vi "Continuous Output.vi"() -> ()   [LabVIEW 2014]
doc: "This example demonstrates how to continuously re-generate analog output data from a buffer in your computer's memory.\n\nRefer to your device documentation for pinouts and hardware capabilities."
uses:
  <vilib>/Utility/error.llb/DialogType.ctl
  <vilib>/DAQmx/write.llb/DAQmx Write (Analog 1D Wfm NChan NSamp).vi
  <vilib>/DAQmx/create/channels.llb/DAQmx Create Channel (AO-Voltage-Basic).vi
  <vilib>/DAQmx/configure/timing.llb/DAQmx Timing (Sample Clock).vi
  <vilib>/DAQmx/miscellaneous.llb/DAQmx Fill In Error Info.vi
  <resource>/objmgr/daqmx.rc
  <vilib>/measure/NI_MABase.lvlib
panel:
  in  "Output Array":T1(array[cluster])=[{"Waveform Type"=0, "Amplitude"=1.0, "Frequency"=10.0}] {"Frequency" format="%0.2p"; "Amplitude" format="%0.2p"; "Waveform Type" items=["Sine Wave", "Triangle Wave", "Square Wave", "Sawtooth Wave"]}
  in  "Number of Samples":i32=1000
  in  "Stop":bool
  out "Waveform Graph":waveform(dbl)[](graph)=[{"t0"=timestamp(0 s since 1904-01-01), "dt"=0.001, "Y"=[]}]
  in  "Sample Rate":dbl=1000.0
  in  "Sample Clock Source":tag="OnboardClock"
  in  "Max Voltage":dbl=5.0
  in  "Min Voltage":dbl=-5.0
  in  "Physical Channel(s)":tag="Dev1/ao0"
  out "Actual Sample Rate":dbl=1000.0 format="%0.2f"
  # "Channel Settings"
  # "Output"
  # "Timing and Buffer Settings"
  # "Waveform Settings"
  # "The number of elements in the waveform array must equal the number of channels in the task."
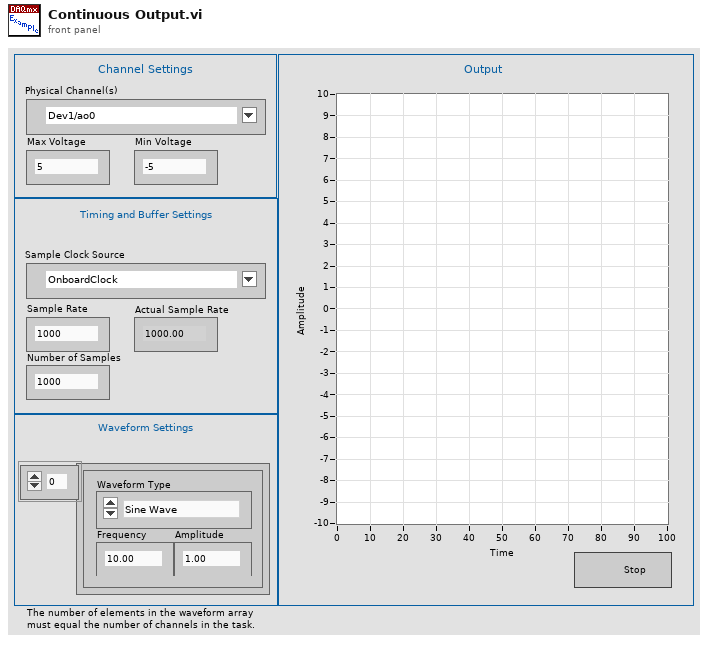
[diagram p1: front panel]
types:
  T1 = cluster{"Waveform Type":u16, "Amplitude":dbl, "Frequency":dbl}[]
  T2 = typedef "DialogType.ctl" = u16
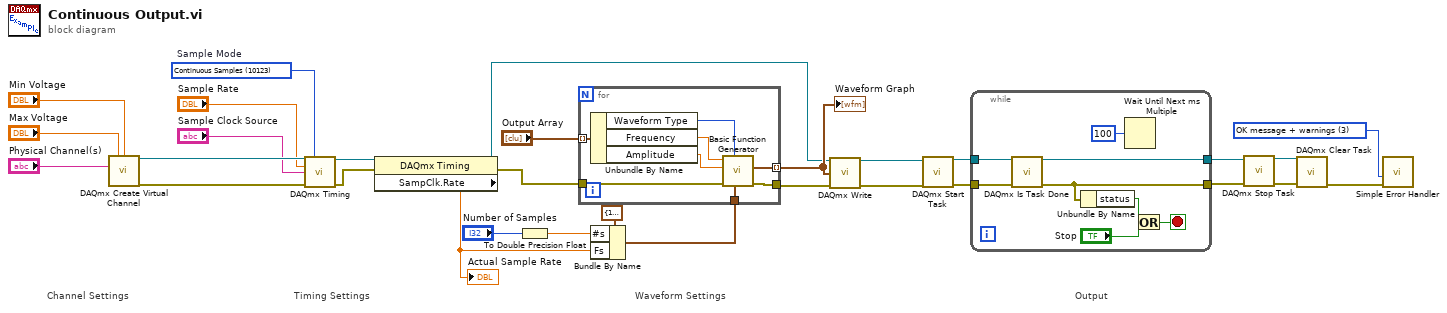
[diagram p0: block diagram]
diagram:
  w3 = T2 3 items=["no dialog", "OK message", "continue or stop message", "OK message + warnings", "continue/stop + warnings"] ("type of dialog (OK msg:1)")
  w28 = 10123 items=["Finite Samples"=10178, "Continuous Samples"=10123, "Hardware Timed Single Point"=12522]  # Sample Mode
  # "Output"
  # "Waveform Settings"
  # "Timing Settings"
  # "Channel Settings"
  n1 = call-poly <vilib>:"DAQmx Create Virtual Channel.vi"("maximum value"="Max Voltage", "minimum value"="Min Voltage", "physical channels"="Physical Channel(s)") -> ("task out"=w26:refnum<k21>, "error out"=w27:errorcluster)  [unwired: 11 in]
  n2 = call-poly <vilib>:"DAQmx Timing.vi"("task/channels in"=w26, "sample mode"=w28, "rate"="Sample Rate", "source"="Sample Clock Source", "error in"=w27) -> ("task out"=w30:refnum<k21>, "error out"=w29:errorcluster)  [unwired: 9 in]
  n3 = property class="DAQmx Timing"(reference=w30, error in=w29) -> (reference out=w2:refnum<k21>, error out=w1:errorcluster, "SampClk.Rate"=w16:dbl)
  "Actual Sample Rate" <- w16
  n4 = To Double Precision Float(number="Number of Samples") -> (double precision float=w9:dbl)
  n5 = Bundle By Name(cluster=cluster{"Fs":dbl, "#s":dbl} {"Fs"=1000.0, "#s"=1000.0} ("sampling info"), "#s"=w9, "Fs"=w16) -> (w15:cluster{"Fs":dbl, "#s":dbl})
  n6 = for {
    tunnel: w1 -> [w38]
    tunnel: w15 -> [w37]
    tunnel: [w36] -> w12
    tunnel: "Output Array" -> [w35] mode=indexing
    tunnel: [w31] -> w10 mode=indexing
    n7 = Unbundle By Name(w35) -> ("Waveform Type"=w34:u16, "Frequency"=w33:dbl, "Amplitude"=w32:dbl)
    n8 = call <vilib>:"Basic Function Generator.vi"("sampling info"=w37, "signal type"=w34, "error in (no error)"=w38, "amplitude"=w32, "frequency"=w33) -> ("error out"=w36:errorcluster, "signal out"=w31:waveform(dbl))  [unwired: 4 in, 1 out]
  }
  "Waveform Graph" <- w10
  n9 = call-poly <vilib>:"DAQmx Write.vi"("task/channels in"=w2, "data"=w10, "error in"=w12) -> ("task out"=w14:refnum<k21>, "error out"=w13:errorcluster)  [unwired: 10 in, 1 out]
  n10 = call <vilib>:"DAQmx Start Task.vi"("task/channels in"=w14, "error in"=w13) -> ("task out"=w25:refnum<k21>, "error out"=w24:errorcluster)  [unwired: 12 in]
  n11 = while {
    tunnel: w25 -> [w46]
    tunnel: w24 -> [w45]
    tunnel: [w42] -> w4
    tunnel: [w43] -> w5
    stop <- w44 stop-if-true
    n12 = call <vilib>:"DAQmx Is Task Done.vi"("task/channels in"=w46, "error in"=w45) -> ("task out"=w43:refnum<k21>, "error out"=w42:errorcluster)  [unwired: 11 in, 1 out]
    n13 = Unbundle By Name(w42) -> ("status"=w41:bool)
    n14 = Wait Until Next ms Multiple(millisecond multiple=u32 100) -> ()  [unwired: 1 out]
    n15 = Or(x=w41, y="Stop") -> (x .or. y?=w44:bool)
  }
  n16 = call <vilib>:"DAQmx Stop Task.vi"("task/channels in"=w5, "error in"=w4) -> ("task out"=w7:refnum<k21>, "error out"=w6:errorcluster)  [unwired: 12 in]
  n17 = call <vilib>:"DAQmx Clear Task.vi"("task in"=w7, "error in"=w6) -> ("error out"=w23:errorcluster)  [unwired: 13 in]
  n18 = call <vilib>:"Simple Error Handler.vi"("type of dialog (OK msg:1)"=w3, "error in (no error)"=w23) -> ()  [unwired: 3 in, 5 out]
